vi "TL_scan_single_step.vi"(4 "Display?":bool, 5 "error in":errorcluster, 6 "Pulse length Ton (s)":sgl=0.01, 7 "image #":i32, 8 "queue CAMERA":refnum<queue>) -> (0 "error out":errorcluster)   [LabVIEW 2015]
uses:
  CONTROLS/Q_camera_element.ctl
  GLOBAL/Global_ABORT.vi
  GLOBAL/Global_CAMERA.vi
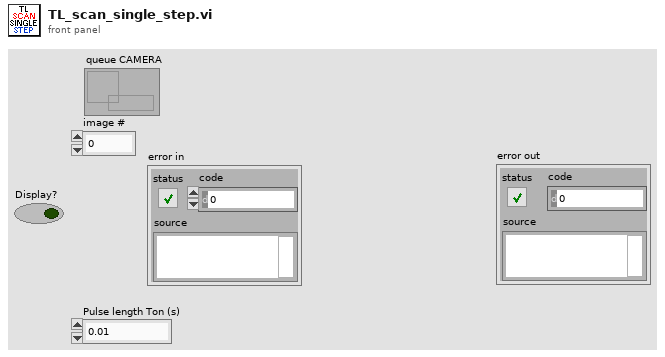
[diagram p1: front panel]
types:
  T1 = cluster{"Pulse length Ton (s)":dbl, "image #":i32, "Display?":bool}
  T2 = typedef "Q_camera_element.ctl" = cluster{"variant":variant, "Instruction":enum16{"CAMERA_idle", "CAMERA_initialize", "CAMERA_error", "CAMERA_security_stop", "CAMERA_not_acquiring", "CAMERA_acquiring", "CAMERA_start_acquiring", "CAMERA_stop_acquiring", "CAMERA_change_exposure", "CAMERA_define_ROI", "CAMERA_cooler", "CAMERA_acquire_movie", "CAMERA_init_scan", "CAMERA_check_new_scan_image", "CAMERA_close_scan", "CAMERA_init_merFISH", "CAMERA_start_acquiring_merFISH", "CAMERA_close_scan_merFISH", "CAMERA_close_merFISH", "CAMERA_init_TL", "CAMERA_start_acquiring_TL", "CAMERA_stop_acquiring_TL", "CAMERA_close_TL", "CAMERA_STOP"}}
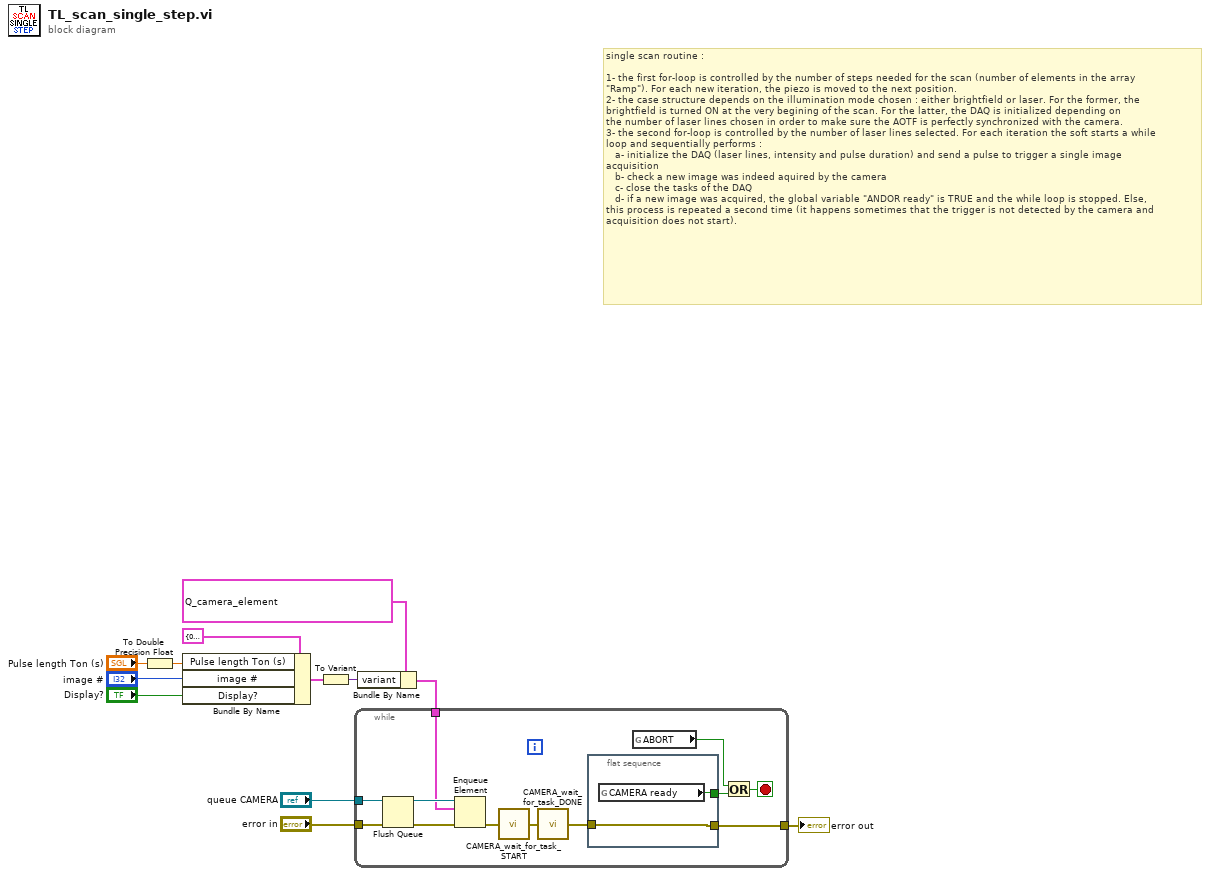
[diagram p0: block diagram]
diagram:
  # "single scan routine :\n\n1- the first for-loop is controlled by the number of steps needed for the scan (number of elements in the array\n\"Ramp\"). For each new iteration, the piezo is moved to the next position.\n2- the case structure depends on the illumination mode chosen : either brightfield or laser. For the former, the\nbrightfield is turned ON at the very begining of the scan. For the latter, the DAQ is initialized depending on\nthe number of laser lines chosen in order to make sure the AOTF is perfectly synchronized with the camera.\n3- the second for-loop is controlled by the number of laser lines selected. For each iteration the soft starts a while\nloop and sequentially performs :\n   a- initialize the DAQ (laser lines, intensity and pulse duration) and send a pulse to trigger a single image\nacquisition\n   b- check a new image was indeed aquired by the camera\n   c- close the tasks of the DAQ\n   d- if a new image was acquired, the global variable \"ANDOR ready\" is TRUE and the while loop is stopped. Else, \nthis process is repeated a second time (it happens sometimes that the trigger is not detected by the camera and\nacquisition does not start)."
  n1 = To Double Precision Float(number="Pulse length Ton (s)") -> (double precision float=w3:dbl)
  n2 = Bundle By Name(cluster=T1 {"Pulse length Ton (s)"=0.0, "image #"=0, "Display?"=FALSE} ("output cluster"), "Pulse length Ton (s)"=w3, "image #"="image #", "Display?"="Display?") -> (w2:T1)
  n3 = To Variant(anything=w2) -> (Variant=w12:variant)
  n4 = Bundle By Name(cluster=T2 {"variant"=variant, "Instruction"=enum."CAMERA_check_new_scan_image"} ("element"), "variant"=w12) -> (w11:T2)
  n5 = while {
    tunnel: "error in" -> [w14]
    tunnel: "queue CAMERA" -> [w16]
    tunnel: w11 -> [w13]
    tunnel: [w24] -> w9
    stop <- w23 stop-if-true
    n6 = Flush Queue(queue=w16, error in (no error)=w14) -> (queue out=w20:refnum<queue>, error out=w19:errorcluster)  [unwired: 1 out]
    n7 = Enqueue Element(queue=w20, element=w13, error in (no error)=w19) -> (error out=w18:errorcluster)  [unwired: 1 in, 2 out]
    n8 = call "CAMERA_wait_for_task_START.vi"("error in"=w18) -> ("error out"=w17:errorcluster)
    n9 = call "CAMERA_wait_for_task_DONE.vi"("error in"=w17) -> ("error out"=w15:errorcluster)
    n10 = flat-sequence {
      tunnel: [w25] -> w22
      tunnel: [w26] -> w24
      tunnel: w15 -> [w26]
      frame #0 {
        n11 = global read "Global_CAMERA.vi" "CAMERA ready"() -> (w25:bool)
      }
    }
    n12 = global read "Global_ABORT.vi" "ABORT"() -> (w21:bool)
    n13 = Or(x=w21, y=w22) -> (x .or. y?=w23:bool)
  }
  "error out" <- w9
